vi "run.vi"(8 "error in (no error)":errorcluster, 11 "StimulatorDL090727DAQmx in":refnum<class "StimulatorDL090727Writer.lvclass">) -> (0 "error out":errorcluster, 3 "StimulatorDL090727DAQmx out":refnum<class "StimulatorDL090727Writer.lvclass">)   [LabVIEW 2010, in "StimulatorDL090727Writer.lvclass"]
uses:
  StimulatorDL090727Writer.lvclass
  pattern_enum.ctl
  common/xcontrols/XSettings/XSettings/XSettings.xctl
  common/classes/GenericComponent/GenericComponent/GenericComponent.lvclass
  main/labview_source/controls/undock_button.ctl
  StimulatorDL090727Writer.lvclass/StimulatorDL090727Writer.ctl
  StimulatorDL090724Scaffold/StimulatorDL090724Scaffold/Stimulator090724Scaffold.lvclass
  common/classes/ErrorController/ErrorController/class_data.vi
  GenericStimulator/GenericStimulator/GenericStimulator.lvclass
  common/classes/ErrorController/ErrorController/ErrorController.lvclass
panel:
  in  "button:undock":T1
  in  "Tab Control":enum32{"User", "Debug", "About"}(tab)
  in  "duration":dbl[unit]=1.0
  in  "offset":dbl[unit]
  in  "duty cycle":dbl[unit]
  in  "repetitions":i32=1
  in  "type":T2
  in  "frequency":dbl[unit]=1.0
  in  "amplitude":dbl=1.0
  in  "settings":refnum<class "GenericComponent.lvclass">(xcontrol)
  out "stop?":bool
  out "event loop error":errorcluster
  # "application"
  # "pattern"
  # "StimulatorDL090727DAQmx\n\nImplemented by:\nDominik Langer, University of Zurich"
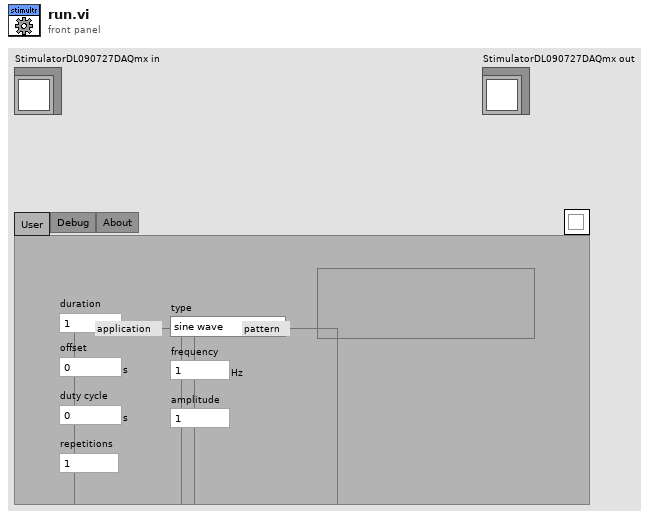
[diagram p1: front panel]
types:
  T1 = typedef "undock_button.ctl" = bool
  T2 = typedef "StimulatorDL090727Writer.lvclass/pattern_enum.ctl" = enum16{"sine wave", "square"}
  T3 = typedef "GenericToplevelComponent.lvclass/common_trigger_enum.ctl" = enum16{"NULL", "initialise", "terminate", "fetch command", "fetch data", "attach observer", "register as observer", "detach observer", "acknowledge", "start", "stop", "sweep started", "sweep finished", "experiment started", "experiment stopped"}
  T4 = enum8{"Enabled", "Disabled", "Disabled and Grayed Out"}
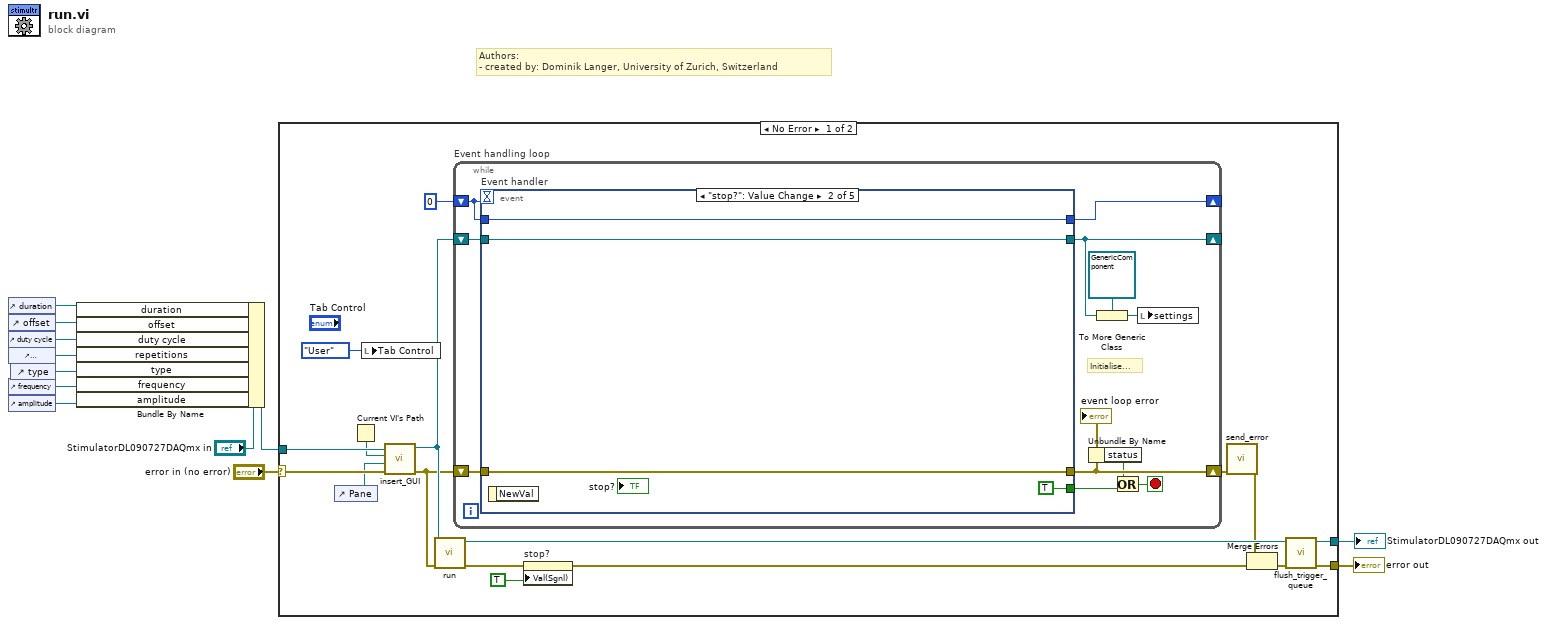
[diagram p0: block diagram]
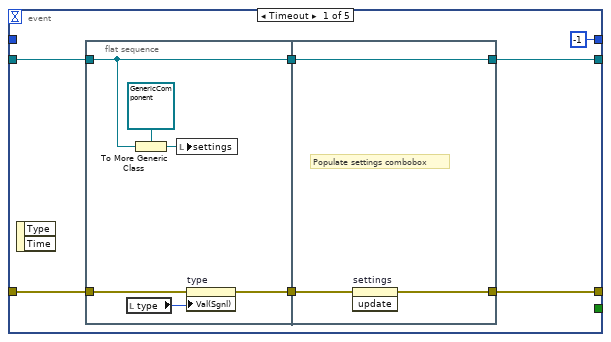
[diagram p2: hidden frame]
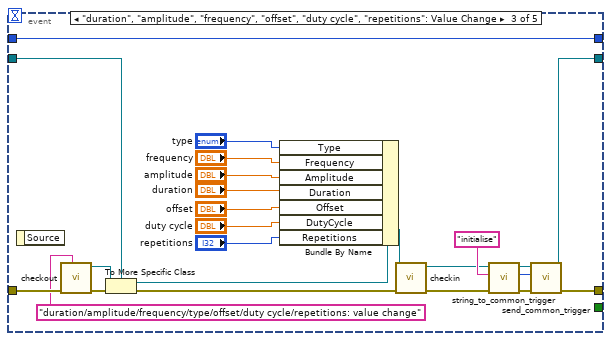
[diagram p3: hidden frame]
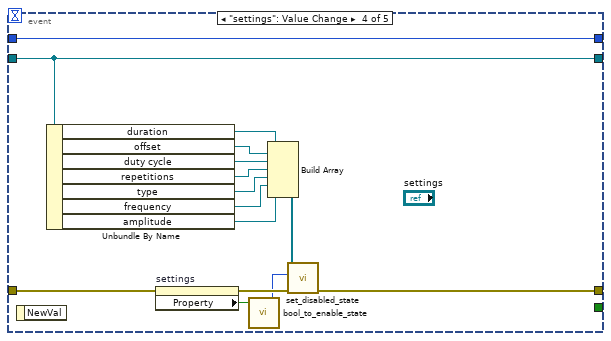
[diagram p4: hidden frame]
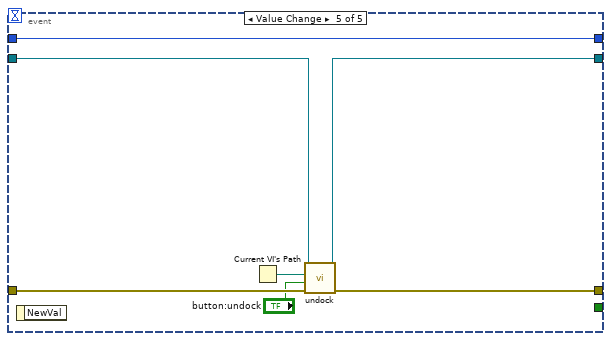
[diagram p5: hidden frame]
diagram:
  # "Authors: \n- created by: Dominik Langer, University of Zurich, Switzerland"
  n1 = control-ref of="duration"() -> (w7:refnum<vi>)
  n2 = control-ref of="offset"() -> (w6:refnum<vi>)
  n3 = control-ref of="duty cycle"() -> (w5:refnum<vi>)
  n4 = control-ref of="repetitions"() -> (w4:refnum<vi>)
  n5 = control-ref of="frequency"() -> (w2:refnum<vi>)
  n6 = control-ref of="amplitude"() -> (w1:refnum<vi>)
  n7 = control-ref of="type"() -> (w3:refnum<vi>)
  n8 = Bundle By Name(cluster="StimulatorDL090727DAQmx in", "duration"=w7, "offset"=w6, "duty cycle"=w5, "repetitions"=w4, "type"=w3, "frequency"=w2, "amplitude"=w1) -> (w8:refnum<class "StimulatorDL090727Writer.lvclass">)
  n9 = case shown="No Error" "error in (no error)" {
    selector: "error in (no error)" -> [w23 w108]
    tunnel: w8 -> [w25 w107]
    tunnel: [w15 w108] -> w11
    tunnel: [w16 w107] -> w10
    frame No Error {
      n10 = control-ref of="Pane"() -> (w20:refnum<vi>)
      n11 = Current VI's Path() -> (path=w21:path)
      n12 = local write "Tab Control"(enum32{"User", "Debug", "About"}."User" ("Tab Control")) -> ()
      n13 = call-dynamic "insert_GUI.vi"("error in (no error)"=w23, "Pane"=w20, "VI path"=w21, "GenericComponent in"=w25) -> ("error out"=w22:errorcluster, "GenericComponent out"=w24:refnum<class "StimulatorDL090727Writer.lvclass">)  [unwired: 6 in]
      n14 = call-parent "run.vi"("error in (no error)"=w22, "Stimulator090724Scaffold in"=w24) -> ("error out"=w27:errorcluster, "Stimulator090724Scaffold out"=w17:refnum<class "StimulatorDL090727Writer.lvclass">)  [unwired: 8 out]
      n15 = while "Event handling loop" {
        shift-right: [w33] -> w14
        shift-left: w22 -> [w40]
        shift-right: [w37] -> _
        shift-left: 0 -> [w38]
        shift-right: [w34] -> _
        shift-left: w24 -> [w39]
        stop <- w30 stop-if-true
        # "Initialise..."
        n16 = event "Event handler" shown="[1] \"stop?\": Value Change" {
          selector: _ -> [_ _ _ _ _]
          dyn-events: _ -> [_ _ _ _ _]
          timeout: w38 -> [_ _ _ _ _]
          tunnel: w40 -> [w46 w60 w83 w91 w105]
          tunnel: [w41 w60 w74 w90 w104] -> w33
          tunnel: w39 -> [w45 w57 w80 w88 w101]
          tunnel: [-1 w59 w84 w99 w106] -> w37
          tunnel: w38 -> [_ w59 w84 w99 w106]
          tunnel: [_ TRUE _ _ _] -> w31
          tunnel: [w42 w57 w67 w88 w100] -> w34
          event Timeout {
            n17 = event-data() -> ()  [unwired: 3 out]
            n18 = flat-sequence {
              tunnel: w46 -> [w52]
              tunnel: w45 -> [w48]
              tunnel: [w51] -> w44
              tunnel: [w48] -> w43
              tunnel: [w54] -> w41
              tunnel: w44 -> [w55]
              tunnel: w43 -> [w56]
              tunnel: [w56] -> w42
              frame #0 {
                n19 = local read "type"() -> (w53:T2)
                n20 = To More Generic Class(target class=refnum<class "GenericComponent.lvclass"> refnum ("GenericComponent.lvclass"), reference=w48) -> (generic class reference=w50:refnum<class "GenericComponent.lvclass">)
                n21 = local write "settings"(w50) -> ()
                n22 = property on="type" class="Enum (strict)"(error in=w52, "Val(Sgnl)"=w53) -> (error out=w51:errorcluster)  [unwired: 1 in, 1 out]
              }
              frame #1 {
                # "Populate settings combobox"
                n23 = invoke on="settings" class="XSettings (strict)" method="update"(error in=w55) -> (error out=w54:errorcluster)  [unwired: 2 in, 2 out]
              }
            }
          }
          event "stop?": Value Change {
            n24 = event-data() -> ()  [unwired: 2 out]
          }
          event "duration", "amplitude", "frequency", "offset", "duty cycle", "repetitions": Value Change {
            n25 = event-data() -> ()  [unwired: 2 out]
            n26 = call "checkout.vi"("locked by?"="duration/amplitude/frequency/type/offset/duty cycle/repetitions: value change", "error in (no error)"=w83) -> ("error out"=w82:errorcluster, "GenericStimulator out"=w81:refnum<class "GenericStimulator.lvclass">)  [unwired: 8 out]
            n27 = To More Specific Class(target class=w80, reference=w81, error in=w82) -> (specific class reference=w75:refnum<class "StimulatorDL090727Writer.lvclass">, error out=w72:errorcluster)
            n28 = Bundle By Name(cluster=w75, "Type"="type", "Frequency"="frequency", "Amplitude"="amplitude", "Duration"="duration", "Offset"="offset", "DutyCycle"="duty cycle", "Repetitions"="repetitions") -> (w73:refnum<class "StimulatorDL090727Writer.lvclass">)
            n29 = call-dynamic "checkin.vi"("error in (no error)"=w72, "GenericStimulator in"=w73) -> ("error out"=w62:errorcluster, "GenericStimulator out"=w64:refnum<class "StimulatorDL090727Writer.lvclass">)  [unwired: 8 in]
            n30 = call-dynamic "string_to_common_trigger.vi"("error in (no error)"=w62, "trigger string"="initialise", "GenericToplevelComponent in"=w64) -> ("error out"=w61:errorcluster, "trigger"=w66:T3, "GenericToplevelComponent out"=w63:refnum<class "StimulatorDL090727Writer.lvclass">)  [unwired: 6 in]
            n31 = call-dynamic "send_common_trigger.vi"("error in (no error)"=w61, "trigger"=w66, "GenericToplevelComponent in"=w63) -> ("error out"=w74:errorcluster, "GenericToplevelComponent out"=w67:refnum<class "StimulatorDL090727Writer.lvclass">)  [unwired: 6 in, 1 out]
          }
          event "settings": Value Change {
            n32 = event-data() -> ()  [unwired: 2 out]
            n33 = Unbundle By Name(w88) -> ("duration"=w98:refnum<vi>, "offset"=w97:refnum<vi>, "duty cycle"=w96:refnum<vi>, "repetitions"=w95:refnum<vi>, "type"=w94:refnum<vi>, "frequency"=w93:refnum<vi>, "amplitude"=w92:refnum<vi>)
            n34 = property on="settings" class="XSettings (strict)"(error in=w91) -> (error out=w87:errorcluster, "Property"=w86:bool)  [unwired: 1 in, 1 out]
            n35 = call "bool_to_enable_state.vi"("boolean in"=w86) -> ("enabled status out"=w85:T4)  [unwired: 4 in]
            n36 = Build Array(w98, w97, w96, w95, w94, w93, w92) -> (w89:refnum<vi>[])
            n37 = call "set_disabled_state.vi"("error in"=w87, "status in"=w85, "control references"=w89) -> ("error out"=w90:errorcluster)  [unwired: 8 in]
          }
          event Value Change {
            n38 = event-data() -> ()  [unwired: 2 out]
            n39 = Current VI's Path() -> (path=w102:path)
            n40 = call-dynamic "undock.vi"("error in (no error)"=w105, "undock?"="button:undock", "VI path"=w102, "component in"=w101) -> ("error out"=w104:errorcluster, "component out"=w100:refnum<class "StimulatorDL090727Writer.lvclass">)  [unwired: 6 in]
          }
        }
        "event loop error" <- w33
        n41 = Unbundle By Name(w33) -> ("status"=w32:bool)
        n42 = To More Generic Class(target class=refnum<class "GenericComponent.lvclass"> refnum ("GenericComponent.lvclass"), reference=w34) -> (generic class reference=w35:refnum<class "GenericComponent.lvclass">)
        n43 = Or(x=w32, y=w31) -> (x .or. y?=w30:bool)
        n44 = local write "settings"(w35) -> ()
      }
      n45 = property on="stop?" class="Bool (strict)"(error in=w27, "Val(Sgnl)"=TRUE) -> (error out=w26:errorcluster)  [unwired: 1 in, 1 out]
      n46 = call "send_error.vi"("error in (no error)"=w14) -> ("error out"=w13:errorcluster)  [unwired: 10 in]
      n47 = Merge Errors(w13, w26) -> (w18:errorcluster)
      n48 = call-dynamic "flush_trigger_queue.vi"("error in (no error)"=w18, "GenericToplevelComponent in"=w17) -> ("error out"=w15:errorcluster, "GenericToplevelComponent out"=w16:refnum<class "StimulatorDL090727Writer.lvclass">)  [unwired: 8 in]
    }
    frame Error {
    }
  }
  "error out" <- w11
  "StimulatorDL090727DAQmx out" <- w10
